vi "FFT To Spectrum_modified_20190812.vi"(0 "real FFT data":dbl[](array[numeric]), 5 "imaginary FFT data":dbl[](array[numeric]), 9 "sample rate (S/s)":dbl format="%#_6p", 11 "error in (no error)":errorcluster) -> (4 "spectrum out (V)":dbl[](array[numeric]), 6 "TheEugeneHong":dbl[][](array[numeric]), 10 "df (Hz)":dbl, 15 "error out":errorcluster)   [LabVIEW 2018]
doc: "Converts the output of the Fast Fourier Transform (FFT) Express VI to a power or amplitude spectrum. The spectrum is single-sided and scaled."
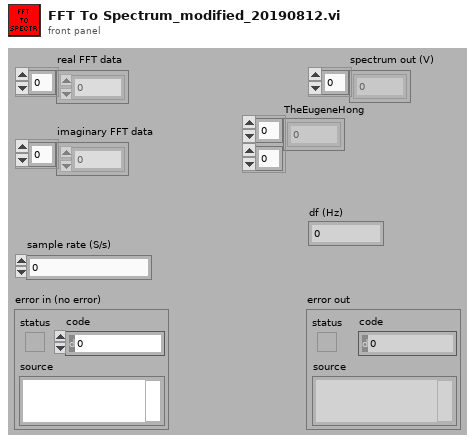
[diagram p1: front panel]
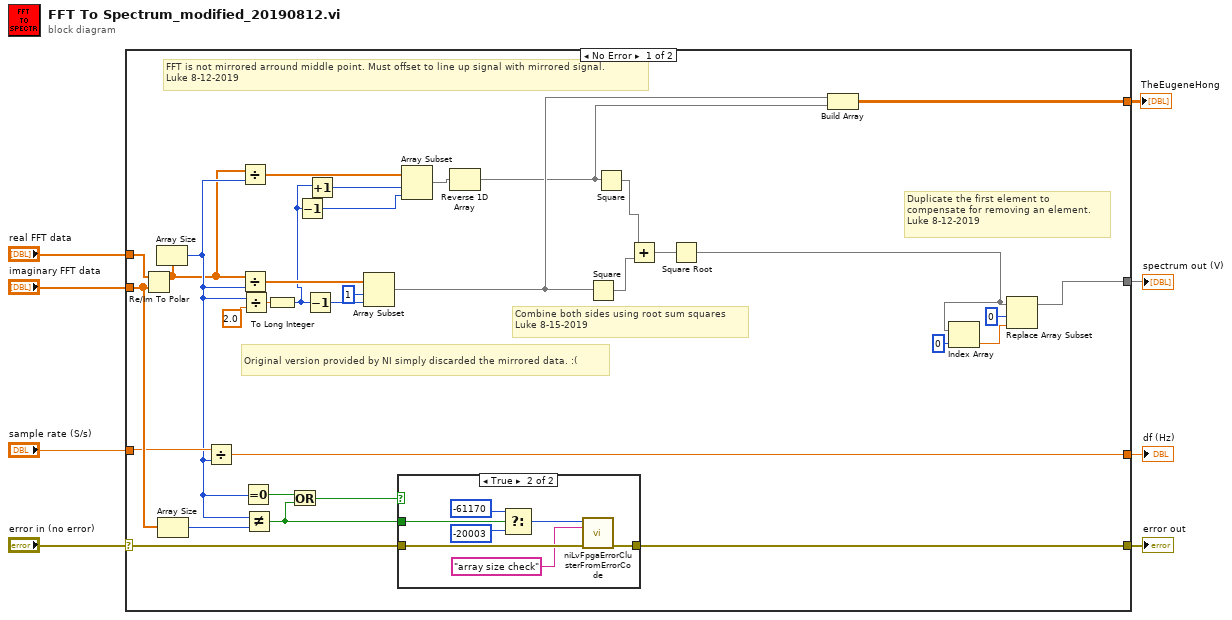
[diagram p0: block diagram]
diagram:
  n1 = case shown="No Error" "error in (no error)" {
    selector: "error in (no error)" -> [w33 w50]
    tunnel: "sample rate (S/s)" -> [w36 _]
    tunnel: [w32 w50] -> w7
    tunnel: "real FFT data" -> [w38 _]
    tunnel: "imaginary FFT data" -> [w37 _]
    tunnel: [w35 _] -> w3
    tunnel: [w22 _] -> w2
    tunnel: [w12 _] -> w1
    frame No Error {
      # "Combine both sides using root sum squares\nLuke 8-15-2019"
      # "Duplicate the first element to \ncompensate for removing an element.\nLuke 8-12-2019"
      # "FFT is not mirrored arround middle point. Must offset to line up signal with mirrored signal.\nLuke 8-12-2019"
      # "Original version provided by NI simply discarded the mirrored data. :("
      n2 = Re/Im To Polar(2:w37, 3:w38) -> (1:w10:dbl[])  [unwired: 1 out]
      n3 = Array Size(array=w10) -> (size(s)=w28:i32)
      n4 = Array Size(array=w37) -> (size(s)=w34:i32)
      n5 = Divide(x=w36, y=w28) -> (x/y=w35:dbl)
      n6 = Divide(x=w10, y=w28) -> (x/y=w19:dbl[])
      n7 = Divide(x=w10, y=w28) -> (x/y=w41:dbl[])
      n8 = Divide(x=w28, y=2.0) -> (x/y=w39:dbl)
      n9 = Equal To 0?(x=w28) -> (x = 0?=w31:bool)
      n10 = Not Equal?(x=w28, y=w34) -> (x != y?=w29:bool)
      n11 = To Long Integer(number=w39) -> (32bit integer=w26:i32)
      n12 = Or(x=w31, y=w29) -> (x .or. y?=w30:bool)
      n13 = Decrement(x=w26) -> (x-1=w17:i32)
      n14 = Decrement(x=w26) -> (x-1=w27:i32)
      n15 = Increment(x=w26) -> (x+1=w16:i32)
      n16 = Array Subset(array=w41, index=1, length=w27) -> (w14:dbl[])
      n17 = case shown="True" w30 {
        tunnel: [w42 w49] -> w32
        tunnel: w33 -> [w42 w48]
        tunnel: w29 -> [_ w44]
        frame False {
        }
        frame True {
          n18 = Select(t=-61170 ("error code"), s=w44, f=-20003 ("error code")) -> (s? t:f=w45:i32)
          n19 = call <vilib>:"niLvFpgaErrorClusterFromErrorCode.vi"("error code"=w45, "function name"="array size check" ("L10N_Function Name"), "error in"=w48) -> ("error out"=w49:errorcluster)  [unwired: 4 in, 8 out]
        }
      }
      n20 = Array Subset(array=w19, index=w16, length=w17) -> (w18:dbl[])
      n21 = Reverse 1D Array(array=w18) -> (reversed array=w13:dbl[])
      n22 = Square(x=w14) -> (x^2=w20:dbl[])
      n23 = Square(x=w13) -> (x^2=w15:dbl[])
      n24 = Add(x=w15, y=w20) -> (x+y=w11:dbl[])
      n25 = Square Root(x=w11) -> (sqrt(x)=w9:dbl[])
      n26 = Build Array(w14, w13) -> (w12:dbl[][])
      n27 = Index Array(array=w9, index=0) -> (element=w24:dbl)
      n28 = Replace Array Subset(array=w9, new element=w24, index=0) -> (w22:dbl[])
    }
    frame Error {
    }
  }
  "error out" <- w7
  "df (Hz)" <- w3
  "spectrum out (V)" <- w2
  "TheEugeneHong" <- w1
